vi "Scroll Delta.vi"(8 "error in (no error)":errorcluster, 10 "Delta":i32, 11 "Terminal in":refnum<class "Terminal.lvclass">) -> (0 "error out":errorcluster, 3 "Terminal out":refnum<class "Terminal.lvclass">)   [LabVIEW 2020, in "Terminal.lvlib" / "Terminal.lvclass"]
uses:
  Terminal.lvclass
  Terminal.lvclass/Terminal.ctl
  TermBuffer/TermBuffer.lvclass
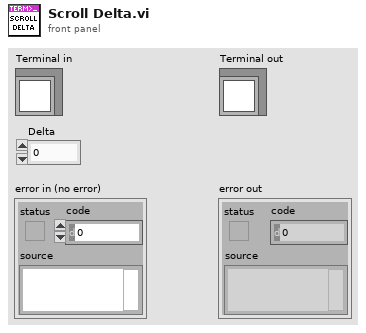
[diagram p1: front panel]
types:
  T1 = typedef "Terminal.lvlib/Terminal.lvclass/Ref Data.ctl" = cluster{"Connection":refnum<class "Connection.lvclass">, "Read Loop Running":bool, "Parse State":T2, "Terminal Options":T7, "Font Metrics":T10, "Scroll":i32, "Close Read Loop":bool}
  T2 = typedef "Terminal.lvlib/Terminal.lvclass/Parse State.ctl" = cluster{"Buffer State":T3, "Cursor":T4, "Attributes":T6}
  T3 = typedef "Terminal.lvlib/Terminal.lvclass/Buffer State.ctl" = cluster{"Sequence":string, "ESC":bool, "Alt Buf":bool}
  T4 = typedef "Terminal.lvlib/Terminal.lvclass/Cursor.ctl" = cluster{"Cur":T5, "Saved":T5}
  T5 = typedef "Terminal.lvlib/Terminal.lvclass/Position.ctl" = cluster{"Row":i32, "Col":i32}
  T6 = typedef "Terminal.lvlib/Text Attributes.ctl" = cluster{"FG":u32, "BG":u32, "Bold":bool, "Italic":bool, "Underline":bool, "Strike":bool, "Inverse":bool}
  T7 = typedef "Terminal.lvlib/Terminal Options.ctl" = cluster{"Implied CR with LF":bool, "Local Echo":bool, "Tab Width":i32, "Color Scheme":T8, "Default FG":T9, "Default BG":T9, "History Length":i32, "Font Face":string, "Font Size":i16, "Rows":i32, "Cols":i32}
  T8 = typedef "Terminal.lvlib/Color Scheme.ctl" = cluster{"Black":u32, "Red":u32, "Green":u32, "Yellow":u32, "Blue":u32, "Magenta":u32, "Cyan":u32, "White":u32, "Bright Black":u32, "Bright Red":u32, "Bright Green":u32, "Bright Yellow":u32, "Bright Blue":u32, "Bright Magenta":u32, "Bright Cyan":u32, "Bright White":u32}
  T9 = typedef "Terminal.lvlib/Color.ctl" = i8
  T10 = typedef "Terminal.lvlib/Terminal.lvclass/Font Metrics.ctl" = cluster{"Width":i16, "Height":i16}
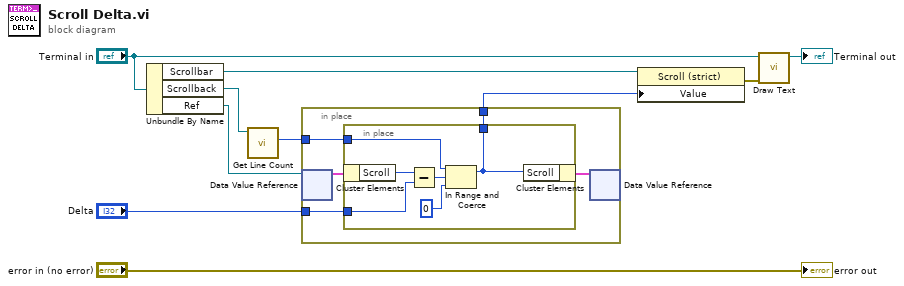
[diagram p0: block diagram]
diagram:
  n1 = Unbundle By Name("Terminal in") -> ("Scrollbar"=w3:refnum<vi>, "Scrollback"=w7:refnum<class "TermBuffer.lvclass">, "Ref"=w9:refnum<data-value>)
  n2 = call "Get Line Count.vi"("TermBuffer in"=w7) -> ("Line Count"=w6:i32)  [unwired: 8 in, 2 out]
  n3 = in-place {
    in-place-border: "Delta" -> [w13]
    in-place-border: w6 -> [w12]
    in-place-border: [w11] -> w2
    n4 = in-place-dvr #1(w9) -> (w15:T1)  [unwired: 1 out]
    n5 = in-place {
      in-place-border: w13 -> [w20]
      in-place-border: w12 -> [w19]
      in-place-border: [w16] -> w11
      n6 = in-place-cluster #2(w15) -> ("Scroll"=w21:i32)
      n7 = Subtract(x=w21, y=w20) -> (x-y=w18:i32)
      n8 = In Range and Coerce(upper limit=w19, x=w18, lower limit=0) -> (coerced(x)=w16:i32)  [unwired: 1 out]
      n9 = in-place-cluster #2("Scroll"=w16) -> (w14:T1)
    }
    n10 = in-place-dvr #1(w14) -> ()  [unwired: 2 out]
  }
  n11 = property class="Scroll (strict)"(reference=w3, "Value"=w2) -> (error out=w1:errorcluster)  [unwired: 1 in, 1 out]
  n12 = call "Draw Text.vi"("error in (no error)"=w1, "Terminal in"="Terminal in") -> ("Terminal out"=→"Terminal out":refnum<class "Terminal.lvclass">)  [unwired: 8 in, 1 out]
  "error out" <- "error in (no error)"
